vi "Computer Write Status.vi"(0 "file path (dialog if empty)":path=path "c:/data/status.csv", 5 "Message":string="Computer Startup", 11 "error in (no error)":errorcluster) -> (15 "error in (no error) 2":errorcluster)   [LabVIEW 2009]
uses:
  <vilib>/Utility/file.llb/Write To Spreadsheet File (string).vi
panel:
  out "Record Written":string[](array[string])
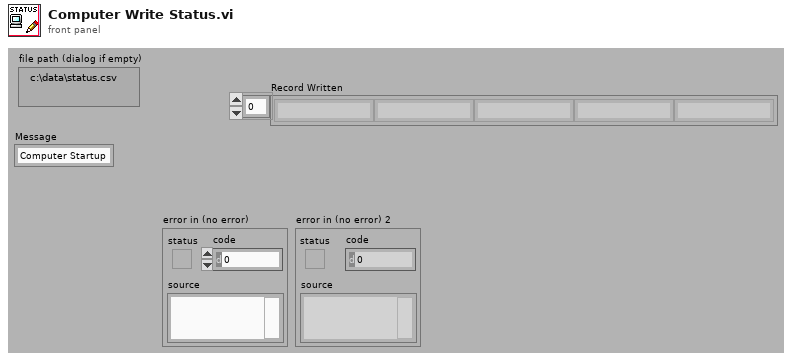
[diagram p1: front panel]
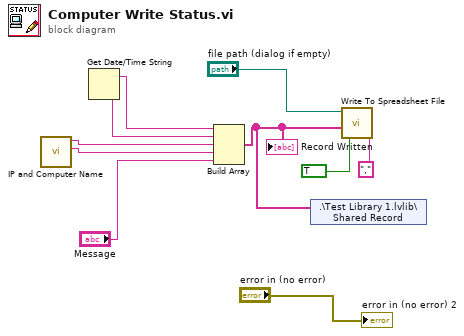
[diagram p0: block diagram]
diagram:
  n1 = call "IP and Computer Name.vi"() -> ("IP Address"=w4:string, "Computer Name"=w5:string)  [unwired: 10 in]
  n2 = Get Date/Time String() -> (date string=w7:string, time string=w6:string)  [unwired: 3 in]
  n3 = Build Array(w7, w6, w5, w4, "Message") -> (w1:string[])
  "Record Written" <- w1
  n4 = shared-variable ".\\Test Library 1.lvlib\\Shared Record"(w1) -> ()  [unwired: 1 in, 1 out]
  n5 = call-poly <vilib>:"Write To Spreadsheet File.vi"("delimiter (\\t)"="," ("delimiter (\\t)"), "append to file? (new file:F)"=TRUE, "1D data"=w1, "file path (dialog if empty)"="file path (dialog if empty)") -> ()  [unwired: 4 in, 1 out]
  "error in (no error) 2" <- "error in (no error)"
